vi "FM Ch Rx Frm Count.vi"(9 "FrmCnt":u32, 10 "Channel":u8, 11 "devId":i32) -> (1 "FrmCnt out":u32, 2 "devId out":i32, 3 "function return":i32)   [LabVIEW 2013, in "CHR34XXX.lvlib"]
doc: "DLL BOOL __stdcall CHR34XXX_FM_Ch_RxMode(IN int devId,IN BYTE Channel,IN BYTE RxMode); DLL BOOL __stdcall CHR34XXX_FM_Ch_RxFrmCount(IN int devId,IN BYTE Channel,OUT DWORD *FrmCnt);"
uses:
  CHR34XXX.lvlib
  CHR34XXX.dll
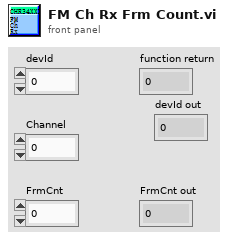
[diagram p1: front panel]
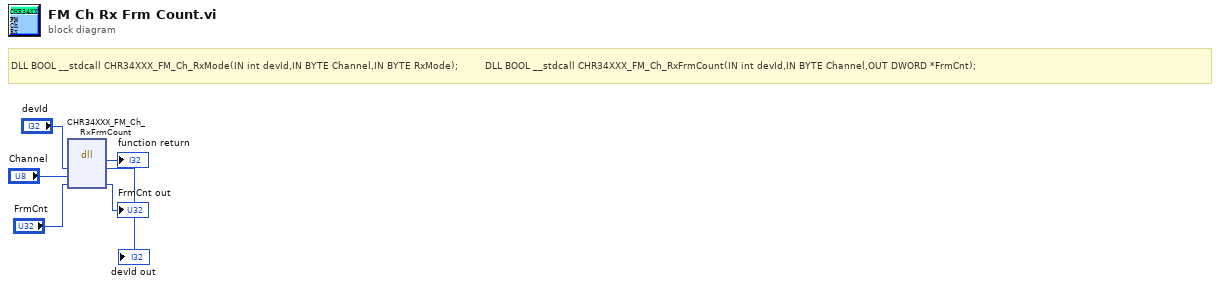
[diagram p0: block diagram]
diagram:
  # "DLL BOOL __stdcall CHR34XXX_FM_Ch_RxMode(IN int devId,IN BYTE Channel,IN BYTE RxMode);         DLL BOOL __stdcall CHR34XXX_FM_Ch_RxFrmCount(IN int devId,IN BYTE Channel,OUT DWORD *FrmCnt);"
  n1 = dll-call lib="C:/Users/Administrator/Desktop/CHR34XXX_lv/lv_lib/CHR34XXX.*" fn="CHR34XXX_FM_Ch_RxFrmCount"("devId"="devId", "Channel"="Channel", "FrmCnt"="FrmCnt") -> (→"function return":i32, "devId"=→"devId out":i32, "FrmCnt"=→"FrmCnt out":u32)  [unwired: 4 in, 2 out]
